vi "sub.vi"(2 "byte count":u32=3) -> (0 "read buffer":string, 1 "x = y?":bool)   [LabVIEW 2014]
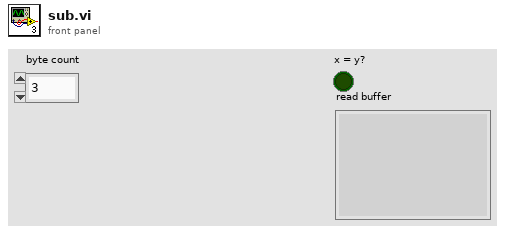
[diagram p1: front panel]
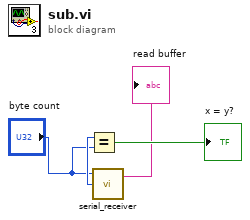
[diagram p0: block diagram]
diagram:
  n1 = call "serial_receiver.vi"("byte count"="byte count") -> ("read buffer"=→"read buffer":string, "return count"=w4:u32)  [unwired: 1 in, 1 out]
  n2 = Equal?(x=w4, y="byte count") -> (x = y?=→"x = y?":bool)
